vi "Read Page Size.vi"(0 "PDF Report":refnum<class "PDF Report Class.lvclass">, 11 "error in (no error)":errorcluster) -> (4 "PDF Report duplicate":refnum<class "PDF Report Class.lvclass">, 6 "Text zone (points)":cluster{"widht":sgl, "height":sgl}={"widht"=612.0, "height"=792.0}, 10 "Page (points)":T1={"Start at page"=1, "Page Size"=0, "Orientation"=enum."Landscape", "widht"=792.0, "height"=72.0, "Margin left"=72.0, "Margin right"=72.0, "Margin top"=72.0, "Margin bottom"=72.0, "X0"=0.0, "X1"=612.0, "Y0"=0.0, "Y1"=792.0} {"Page Size" items=["Custom", "LETTER", "NOTE", "LEGAL", "TABLOID", "EXECUTIVE", "POSTCARD", "A0", "A1", "A2", "A3", "A4", "A5", "A6", "A7", "A8", "A9", "A10", "B0", "B1", "B2", "B3", "B4", "B5", "B6", "B7", "B8", "B9", "B10", "ARCH_E", "ARCH_D", "ARCH_C", "ARCH_B", "ARCH_A", "FLSA", "FLSE", "HALFLETTER", "_11X17", "ID_1", "ID_2", "ID_3", "LEDGER", "CROWN_QUARTO", "LARGE_CROWN_QUARTO", "DEMY_QUARTO", "ROYAL_QUARTO", "CROWN_OCTAVO", "LARGE_CROWN_OCTAVO", "DEMY_OCTAVO", "ROYAL_OCTAVO", "SMALL_PAPERBACK", "PENGUIN_SMALL_PAPERBACK", "PENGUIN_LARGE_PAPERBACK"]}, 15 "error out":errorcluster)   [LabVIEW 2020, in "Exaprom PDF.lvlib"]
doc: "Version 1.0\nDeveloped by Jean-Marc Simard\nCopyright © 2010, Exaprom Inc.\nAll rights reserved.\nLicense: BSD\n\nWith iTextSharp 4.1.6 (http://itextsharp.sourceforge.net)\nunder Mozilla Public License Version 1.1\n(http://www.mozilla.org/MPL/MPL-1.1.html)"
uses:
  <userlib>/labview-PDF-writer-master/Exaprom PDF.lvlib
  <userlib>/labview-PDF-writer-master/LV Class/PDF Report Class/PDF Report Class.lvclass
  <userlib>/labview-PDF-writer-master/Controls/Page Controls/Page dimensions.ctl
  <userlib>/labview-PDF-writer-master/Controls/Page Controls/Page size.ctl
  <userlib>/labview-PDF-writer-master/Controls/Page Controls/Page Orientation.ctl
  C:/Program Files (x86)/National Instruments/LabVIEW 2020/user.lib/labview-PDF-writer-master/DLL/itextsharp.dll
  DLL/itextsharp.dll
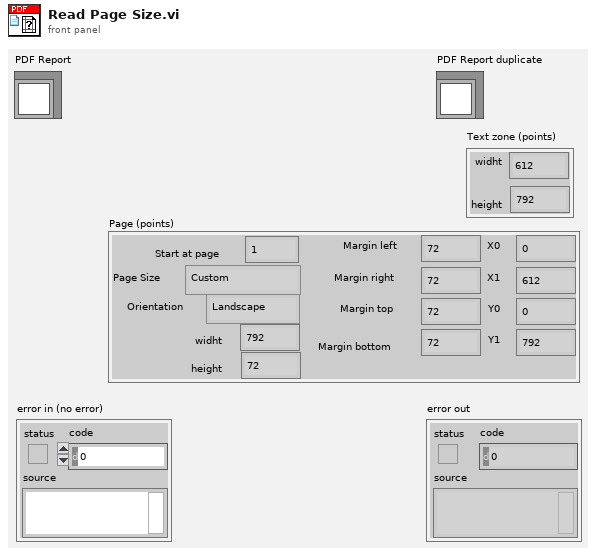
[diagram p1: front panel]
types:
  T1 = typedef "Exaprom PDF.lvlib/Page dimensions.ctl" = cluster{"Start at page":i32, "Page Size":T2, "Orientation":T3, "widht":sgl, "height":sgl, "Margin left":sgl, "Margin right":sgl, "Margin top":sgl, "Margin bottom":sgl, "X0":sgl, "X1":sgl, "Y0":sgl, "Y1":sgl}
  T2 = typedef "Exaprom PDF.lvlib/Page size.ctl" = i32
  T3 = typedef "Exaprom PDF.lvlib/Page Orientation.ctl" = enum16{"Portrait", "Landscape"}
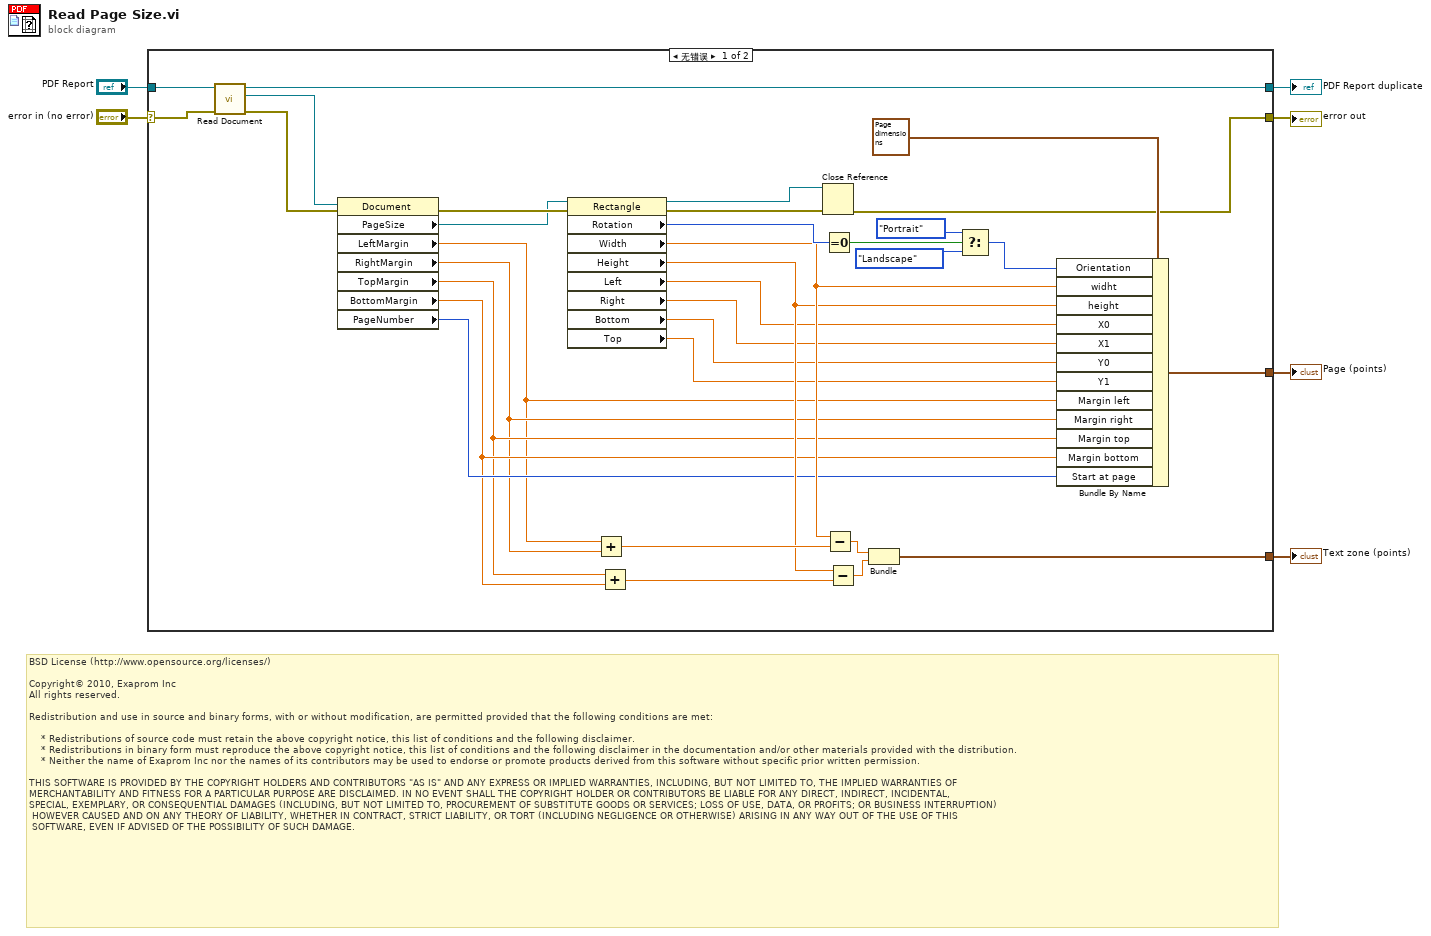
[diagram p0: block diagram]
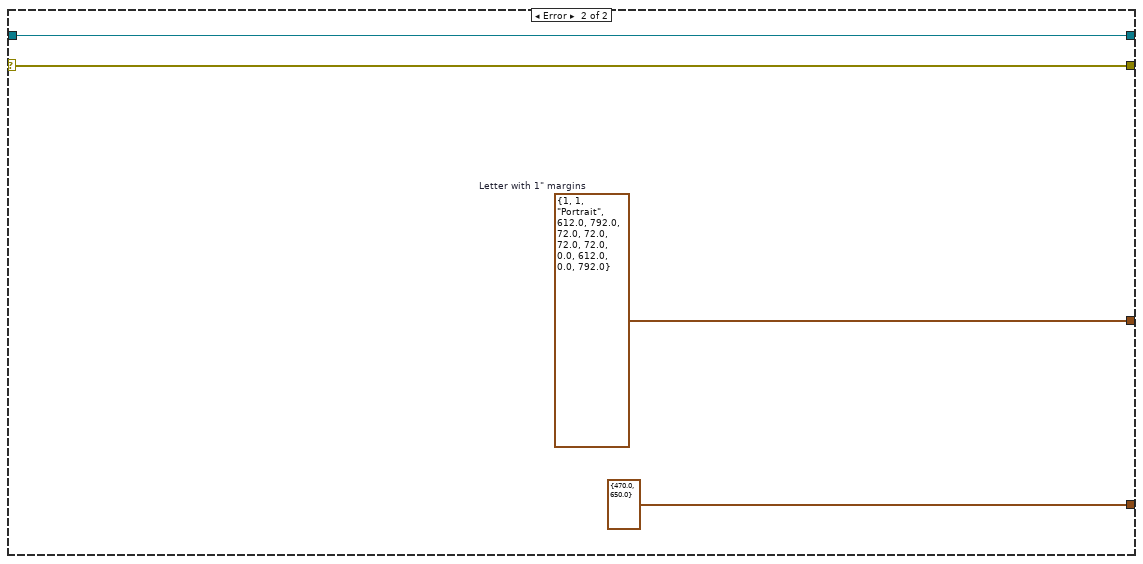
[diagram p2: hidden frame]
diagram:
  # "BSD License (http://www.opensource.org/licenses/)\n\nCopyright© 2010, Exaprom Inc\nAll rights reserved.\n\nRedistribution and use in source and binary forms, with or without modification, are permitted provided that the following conditions are met:\n\n    * Redistributions of source code must retain the above copyright notice, this list of conditions and the following disclaimer.\n    * Redistributions in binary form must reproduce the above copyright notice, this list of conditions and the following disclaimer in the documentation and/or other materials provided with the distribution.\n    * Neither the name of Exaprom Inc nor the names of its contributors may be used to endorse or promote products derived from this software without specific prior written permission.\n\nTHIS SOFTWARE IS PROVIDED BY THE COPYRIGHT HOLDERS AND CONTRIBUTORS \"AS IS\" AND ANY EXPRESS OR IMPLIED WARRANTIES, INCLUDING, BUT NOT LIMITED TO, THE IMPLIED WARRANTIES OF \nMERCHANTABILITY AND FITNESS FOR A PARTICULAR PURPOSE ARE DISCLAIMED. IN NO EVENT SHALL THE COPYRIGHT HOLDER OR CONTRIBUTORS BE LIABLE FOR ANY DIRECT, INDIRECT, INCIDENTAL,\nSPECIAL, EXEMPLARY, OR CONSEQUENTIAL DAMAGES (INCLUDING, BUT NOT LIMITED TO, PROCUREMENT OF SUBSTITUTE GOODS OR SERVICES; LOSS OF USE, DATA, OR PROFITS; OR BUSINESS INTERRUPTION)\n HOWEVER CAUSED AND ON ANY THEORY OF LIABILITY, WHETHER IN CONTRACT, STRICT LIABILITY, OR TORT (INCLUDING NEGLIGENCE OR OTHERWISE) ARISING IN ANY WAY OUT OF THE USE OF THIS\n SOFTWARE, EVEN IF ADVISED OF THE POSSIBILITY OF SUCH DAMAGE."
  n1 = case shown="无错误" "error in (no error)" {
    selector: "error in (no error)" -> [w17 w43]
    tunnel: [w33 w41] -> w6
    tunnel: "PDF Report" -> [w30 w42]
    tunnel: [w27 w43] -> w3
    tunnel: [w19 w42] -> w2
    tunnel: [w20 cluster{sgl, sgl} {470.0, 650.0}] -> w1
    frame No Error {
      n2 = call-dynamic "Read Document.vi"("error in (no error)"=w17, "PDF Report Class in"=w30) -> ("error out"=w16:errorcluster, "Document"=w18:refnum<k24>, "PDF Report Class out"=w19:refnum<class "PDF Report Class.lvclass">)  [unwired: 7 in]
      n3 = property class="Document"(reference=w18, error in=w16) -> (error out=w39:errorcluster, "PageSize"=w38:refnum<k24>, "LeftMargin"=w11:sgl, "RightMargin"=w12:sgl, "TopMargin"=w13:sgl, "BottomMargin"=w14:sgl, "PageNumber"=w15:i32)  [unwired: 1 out]
      n4 = property class="Rectangle"(reference=w38, error in=w39) -> (reference out=w28:refnum<k24>, error out=w29:errorcluster, "Rotation"=w32:i32, "Width"=w26:sgl, "Height"=w24:sgl, "Left"=w10:sgl, "Right"=w9:sgl, "Bottom"=w8:sgl, "Top"=w7:sgl)
      n5 = Add(x=w11, y=w12) -> (x+y=w25:sgl)
      n6 = Add(x=w13, y=w14) -> (x+y=w23:sgl)
      n7 = Close Reference(reference=w28, error in (no error)=w29) -> (error out=w27:errorcluster)
      n8 = Equal To 0?(x=w32) -> (x = 0?=w37:bool)
      n9 = Subtract(x=w26, y=w25) -> (x-y=w22:sgl)
      n10 = Subtract(x=w24, y=w23) -> (x-y=w21:sgl)
      n11 = Bundle(w22, w21) -> (w20:cluster{sgl, sgl})  [unwired: 1 out]
      n12 = Select(t=Page_Orientation."Portrait" ("Orientation"), s=w37, f=Page_Orientation."Landscape" ("Orientation")) -> (s? t:f=w31:T3)
      n13 = Bundle By Name(cluster=T1 {"Start at page"=1, "Page Size"=0, "Orientation"=enum."Landscape", "widht"=792.0, "height"=70.86614, "Margin left"=70.86614, "Margin right"=70.86614, "Margin top"=70.86614, "Margin bottom"=0.0, "X0"=0.0, "X1"=0.0, "Y0"=0.0, "Y1"=0.0} ("Page (points)"), "Orientation"=w31, "widht"=w26, "height"=w24, "X0"=w10, "X1"=w9, "Y0"=w8, "Y1"=w7, "Margin left"=w11, "Margin right"=w12, "Margin top"=w13, "Margin bottom"=w14, "Start at page"=w15) -> (w33:T1)
    }
    frame Error {
      w41 = T1 {"Start at page"=1, "Page Size"=1, "Orientation"=enum."Portrait", "widht"=612.0, "height"=792.0, "Margin left"=72.0, "Margin right"=72.0, "Margin top"=72.0, "Margin bottom"=72.0, "X0"=0.0, "X1"=612.0, "Y0"=0.0, "Y1"=792.0}  # Letter with 1" margins
    }
  }
  "PDF Report duplicate" <- w2
  "Page (points)" <- w6
  "error out" <- w3
  "Text zone (points)" <- w1
